vi "set_params.vi"(8 "error in (no error)":errorcluster caption="entrée d'erreur (pas d'erreur)", 11 "LinearDiscriminantAnalysis.lvclass 2":refnum<class "LinearDiscriminantAnalysis.lvclass">) -> (0 "error out":errorcluster caption="sortie d'erreur", 3 "LinearDiscriminantAnalysis.lvclass":refnum<class "LinearDiscriminantAnalysis.lvclass">)   [LabVIEW 2020, in "LinearDiscriminantAnalysis.lvclass"]
uses:
  LinearDiscriminantAnalysis.lvclass
  LinearDiscriminantAnalysis.lvclass/LinearDiscriminantAnalysis.ctl
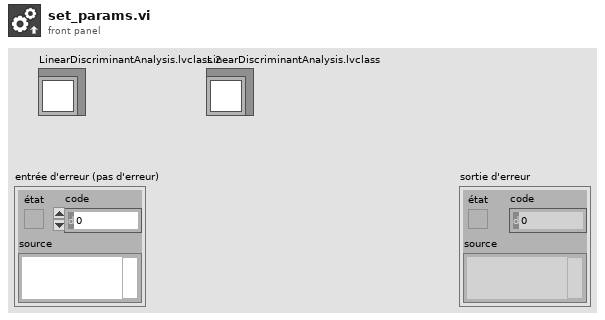
[diagram p1: front panel]
types:
  T1 = typedef "linear_discriminant_analysis_params.ctl" = cluster{"solver":string, "shrinkage":cluster{"shrinkage_type":string, "shrinkage_float":dbl}, "priors":cluster{"priors_type":string, "priors_list":dbl[]}, "n_components":cluster{"n_components_type":string, "n_components_int":dbl}, "store_covariance":bool, "tol":dbl}
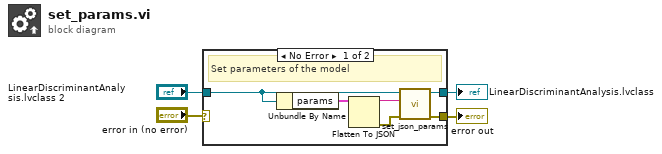
[diagram p0: block diagram]
diagram:
  n1 = case shown="No Error" "error in (no error)" {
    selector: "error in (no error)" -> [_ w12]
    tunnel: [w7 w12] -> w3
    tunnel: [w8 w11] -> w1
    tunnel: "LinearDiscriminantAnalysis.lvclass 2" -> [w5 w11]
    frame No Error {
      # "Set parameters of the model"
      n2 = Unbundle By Name(w5) -> ("params"=w10:T1)
      n3 = Flatten To JSON(anything=w10) -> (JSON string=w9:string, 11:w6:errorcluster)  [unwired: 2 in]
      n4 = call-dynamic "set_json_params.vi"("error in (no error)"=w6, "params"=w9, "Model en entrée"=w5) -> ("error out"=w7:errorcluster, "Model en sortie"=w8:refnum<class "LinearDiscriminantAnalysis.lvclass">)  [unwired: 7 in]
    }
    frame Error {
    }
  }
  "error out" <- w3
  "LinearDiscriminantAnalysis.lvclass" <- w1
